vi "AIM 664 test Import Configuration File (Default Attributes).vi"(8 "error in (no error)":errorcluster, 11 "TestCase in":refnum<class "AIM 664 Import.lvclass">) -> (0 "error out":errorcluster, 3 "TestCase out":refnum<class "AIM 664 Import.lvclass">)   [LabVIEW 2020, in "AIM 664 Import.lvclass"]
uses:
  AIM 664 Import.lvclass
  Shared/Port Session Configuration.ctl
  Shared/board_setup.ctl
  Shared/port_configuration.ctl
  Shared/port_setup.ctl
  Shared/tx_udp_setup.ctl
  Shared/port_tx_udp_comm.ctl
  Shared/frame_parameter.ctl
  Shared/frame_parameter_definition.ctl
  <vilib>/NI/NI VeriStand Encoding and Decoding/Encoding.ctl
  Shared/port_tx_udp_sap.ctl
  Shared/rx_udp_setup.ctl
  Shared/port_rx_udp_comm.ctl
  Shared/port_rx_udp_sap.ctl
  <vilib>/addons/_JKI Toolkits/VI Tester/TestCase.llb/TestCase.lvclass
  <vilib>/NI/VeriStand Custom Device Testing Tools/VeriStandTestUtilities/VeriStandTestUtilities.lvlib
  Import/AIM ARINC 664 Import.lvlib
  <vilib>/NI/NI VeriStand Encoding and Decoding/Encoding and Decoding.lvlib
  C:/Program Files (x86)/National Instruments/LabVIEW 2020/vi.lib/addons/_JKI Toolkits/VI Tester/TestCase.llb/TestCase.lvclass
panel:
  out "x = y?":T1
  out "size(s)":i32
  out "index of element":i32[](array[numeric])
  out "logical AND 6":bool
  out "x = y? 2":bool[](array[boolean])
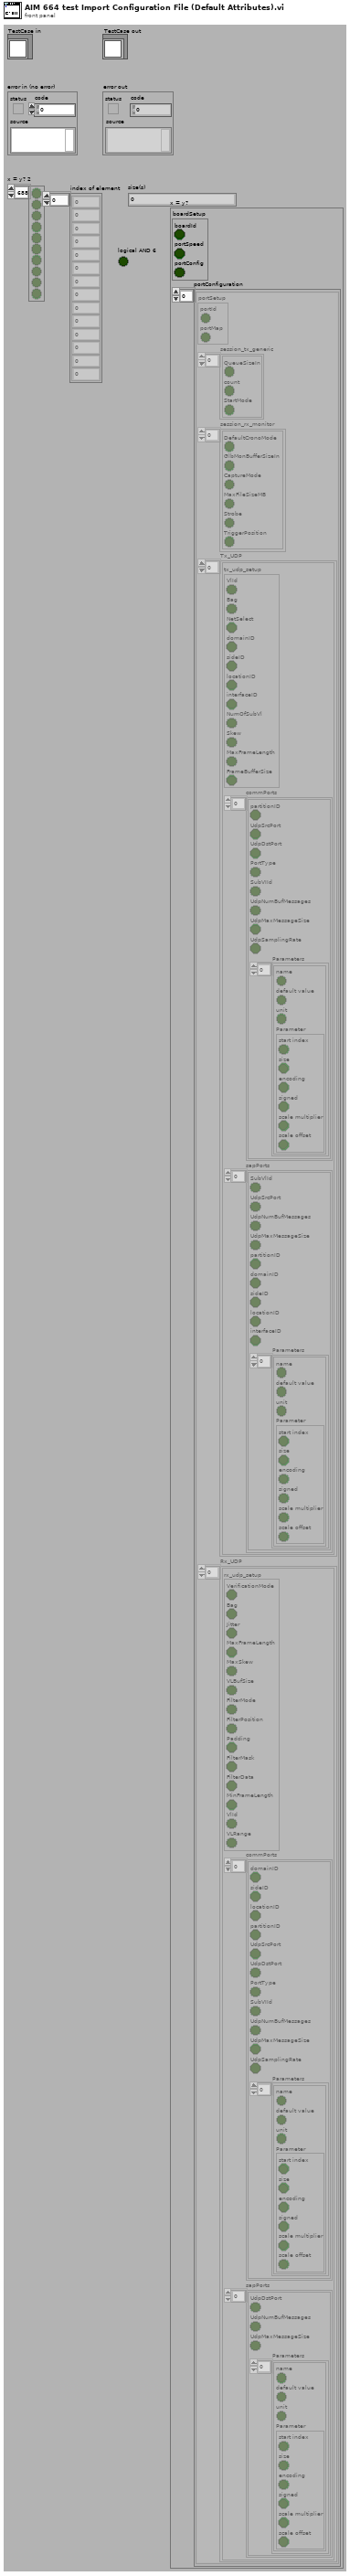
[diagram p1: front panel]
types:
  T1 = cluster{"boardSetup":cluster{"boardId":bool, "portSpeed":bool, "portConfig":bool}, "portConfiguration":cluster{"portSetup":cluster{"portId":bool, "portMap":bool}, "session_tx_generic":cluster{"QueueSizeIn":bool, "count":bool, "StartMode":bool}[], "session_rx_monitor":cluster{"DefaultCronoMode":bool, "GlbMonBufferSizeIn":bool, "CaptureMode":bool, "MaxFileSizeMB":bool, "Strobe":bool, "TriggerPosition":bool}[], "Tx_UDP":cluster{"tx_udp_setup":cluster{"VlId":bool, "Bag":bool, "NetSelect":bool, "domainID":bool, "sideID":bool, "locationID":bool, "interfaceID":bool, "NumOfSubVl":bool, "Skew":bool, "MaxFrameLength":bool, "FrameBufferSize":bool}, "commPorts":cluster{"partitionID":bool, "UdpSrcPort":bool, "UdpDstPort":bool, "PortType":bool, "SubVIId":bool, "UdpNumBufMessages":bool, "UdpMaxMessageSize":bool, "UdpSamplingRate":bool, "Parameters":cluster{"name":bool, "default value":bool, "unit":bool, "Parameter":cluster{"start index":bool, "size":bool, "encoding":bool, "signed":bool, "scale multiplier":bool, "scale offset":bool}}[]}[], "sapPorts":cluster{"SubVlId":bool, "UdpSrcPort":bool, "UdpNumBufMessages":bool, "UdpMaxMessageSize":bool, "partitionID":bool, "domainID":bool, "sideID":bool, "locationID":bool, "interfaceID":bool, "Parameters":cluster{"name":bool, "default value":bool, "unit":bool, "Parameter":cluster{"start index":bool, "size":bool, "encoding":bool, "signed":bool, "scale multiplier":bool, "scale offset":bool}}[]}[]}[], "Rx_UDP":cluster{"rx_udp_setup":cluster{"VerificationMode":bool, "Bag":bool, "Jitter":bool, "MaxFrameLength":bool, "MaxSkew":bool, "VLBufSize":bool, "FilterMode":bool, "FilterPosition":bool, "Padding":bool, "FilterMask":bool, "FilterData":bool, "MinFrameLength":bool, "VlId":bool, "VLRange":bool}, "commPorts":cluster{"domainID":bool, "sideID":bool, "locationID":bool, "partitionID":bool, "UdpSrcPort":bool, "UdpDstPort":bool, "PortType":bool, "SubVIId":bool, "UdpNumBufMessages":bool, "UdpMaxMessageSize":bool, "UdpSamplingRate":bool, "Parameters":cluster{"name":bool, "default value":bool, "unit":bool, "Parameter":cluster{"start index":bool, "size":bool, "encoding":bool, "signed":bool, "scale multiplier":bool, "scale offset":bool}}[]}[], "sapPorts":cluster{"UdpDstPort":bool, "UdpNumBufMessages":bool, "UdpMaxMessageSize":bool, "Parameters":cluster{"name":bool, "default value":bool, "unit":bool, "Parameter":cluster{"start index":bool, "size":bool, "encoding":bool, "signed":bool, "scale multiplier":bool, "scale offset":bool}}[]}[]}[]}[]}
  T2 = typedef "AIM ARINC 664 Import.lvlib/Port Session Configuration.ctl" = cluster{"boardSetup":T3, "portConfiguration":T4[]}
  T3 = typedef "AIM ARINC 664 Import.lvlib/board_setup.ctl" = cluster{"boardId":u32, "portSpeed":u32, "portConfig":u32}
  T4 = typedef "AIM ARINC 664 Import.lvlib/port_configuration.ctl" = cluster{"portSetup":T5, "session_tx_generic":cluster{"QueueSizeIn":u32, "count":i32, "StartMode":i32}[], "session_rx_monitor":cluster{"DefaultCronoMode":u32, "GlbMonBufferSizeIn":u32, "CaptureMode":u32, "MaxFileSizeMB":u32, "Strobe":u32, "TriggerPosition":u32}[], "Tx_UDP":cluster{"tx_udp_setup":T6, "commPorts":T7[], "sapPorts":T11[]}[], "Rx_UDP":cluster{"rx_udp_setup":T12, "commPorts":T13[], "sapPorts":T14[]}[]}
  T5 = typedef "AIM ARINC 664 Import.lvlib/port_setup.ctl" = cluster{"portId":u32, "portMap":u32}
  T6 = typedef "AIM ARINC 664 Import.lvlib/tx_udp_setup.ctl" = cluster{"VlId":i32, "Bag":i32, "NetSelect":i32, "domainID":u8, "sideID":u8, "locationID":u8, "interfaceID":u8, "NumOfSubVl":u16, "Skew":u32, "MaxFrameLength":u32, "FrameBufferSize":u32}
  T7 = typedef "AIM ARINC 664 Import.lvlib/port_tx_udp_comm.ctl" = cluster{"partitionID":u8, "UdpSrcPort":u16, "UdpDstPort":u16, "PortType":enum16{"FDX_UDP_SAMPLING", "FDX_UDP_QUEUING"}, "SubVIId":u32, "UdpNumBufMessages":u32, "UdpMaxMessageSize":u32, "UdpSamplingRate":u32, "Parameters":T8[]}
  T8 = typedef "AIM ARINC 664 Import.lvlib/frame_parameter.ctl" = cluster{"name":string, "default value":dbl, "unit":string, "Parameter":T9}
  T9 = typedef "AIM ARINC 664 Import.lvlib/frame_parameter_definition.ctl" = cluster{"start index":i32, "size":i32, "encoding":T10, "signed":bool, "scale multiplier":dbl, "scale offset":dbl}
  T10 = typedef "Encoding and Decoding.lvlib/Encoding.ctl" = enum16{"BNR", "BCD", "Discrete"}
  T11 = typedef "AIM ARINC 664 Import.lvlib/port_tx_udp_sap.ctl" = cluster{"SubVlId":u8, "UdpSrcPort":u16, "UdpNumBufMessages":u32, "UdpMaxMessageSize":u32, "partitionID":u8, "domainID":u8, "sideID":u8, "locationID":u8, "interfaceID":u8, "Parameters":T8[]}
  T12 = typedef "AIM ARINC 664 Import.lvlib/rx_udp_setup.ctl" = cluster{"VerificationMode":u32, "Bag":u32, "Jitter":u32, "MaxFrameLength":u32, "MaxSkew":u32, "VLBufSize":u32, "FilterMode":u32, "FilterPosition":u32, "Padding":u32, "FilterMask":u32, "FilterData":u32, "MinFrameLength":u32, "VlId":u16, "VLRange":u32}
  T13 = typedef "AIM ARINC 664 Import.lvlib/port_rx_udp_comm.ctl" = cluster{"domainID":u8, "sideID":u8, "locationID":u8, "partitionID":u8, "UdpSrcPort":u16, "UdpDstPort":u16, "PortType":enum16{"FDX_UDP_SAMPLING", "FDX_UDP_QUEUING"}, "SubVIId":u32, "UdpNumBufMessages":u32, "UdpMaxMessageSize":u32, "UdpSamplingRate":u32, "Parameters":T8[]}
  T14 = typedef "AIM ARINC 664 Import.lvlib/port_rx_udp_sap.ctl" = cluster{"UdpDstPort":u16, "UdpNumBufMessages":u32, "UdpMaxMessageSize":u32, "Parameters":T8[]}
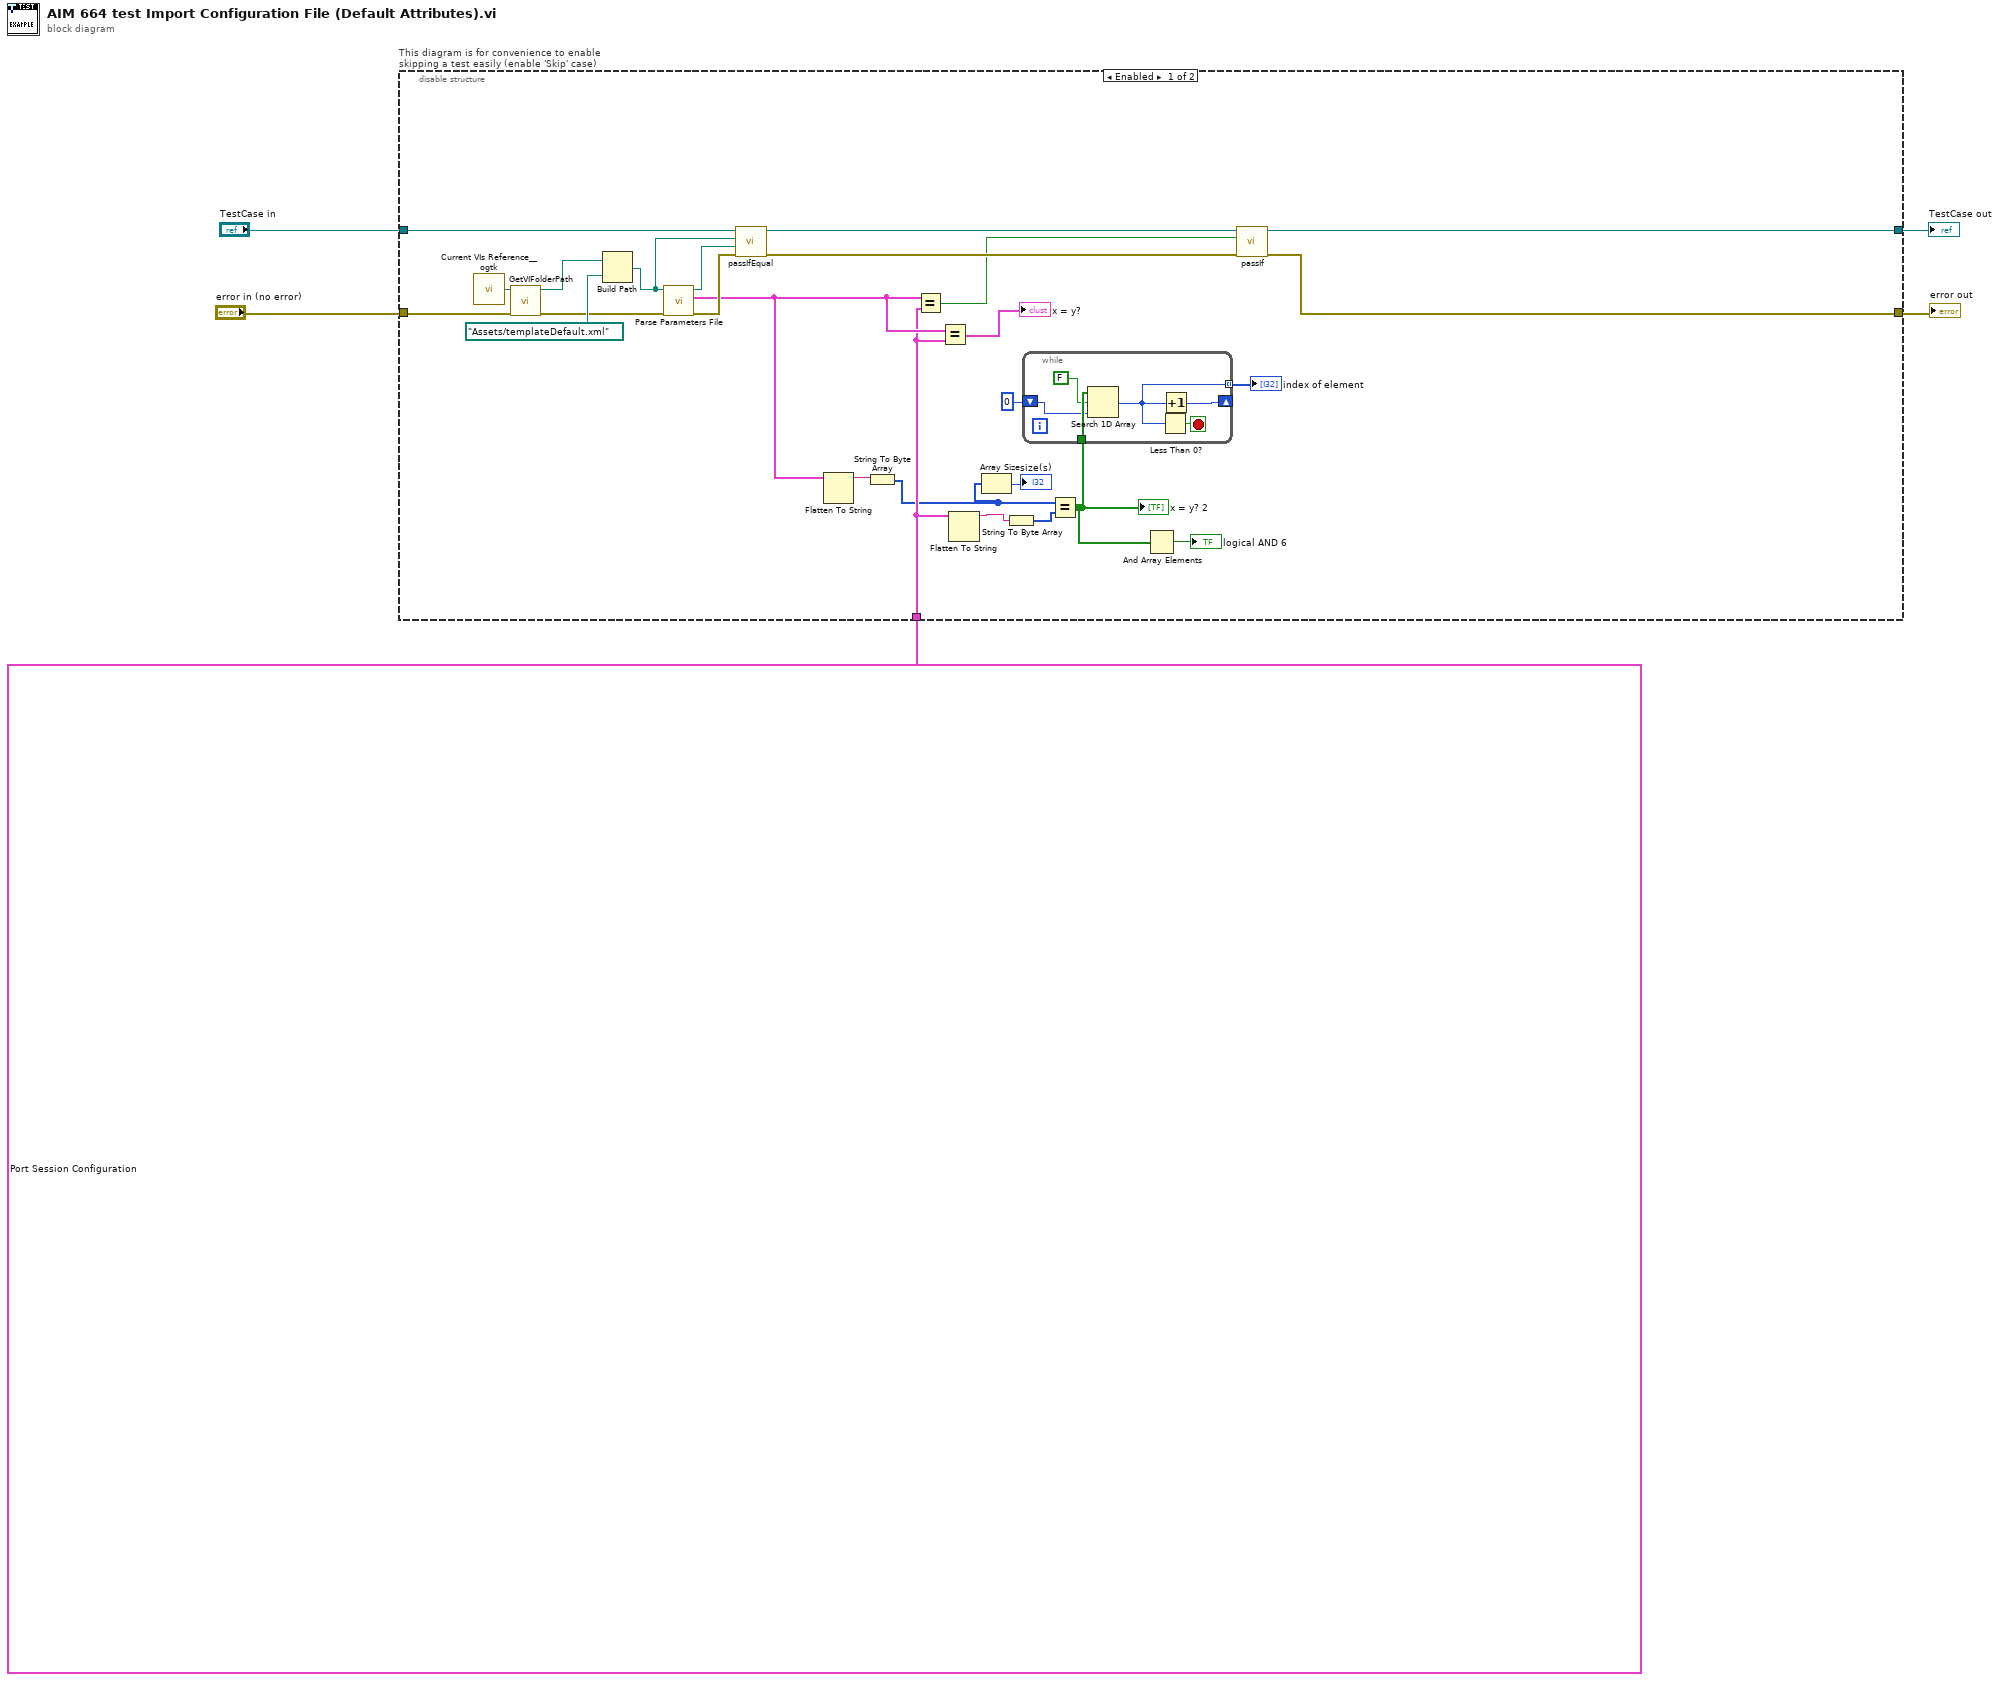
[diagram p0: block diagram]
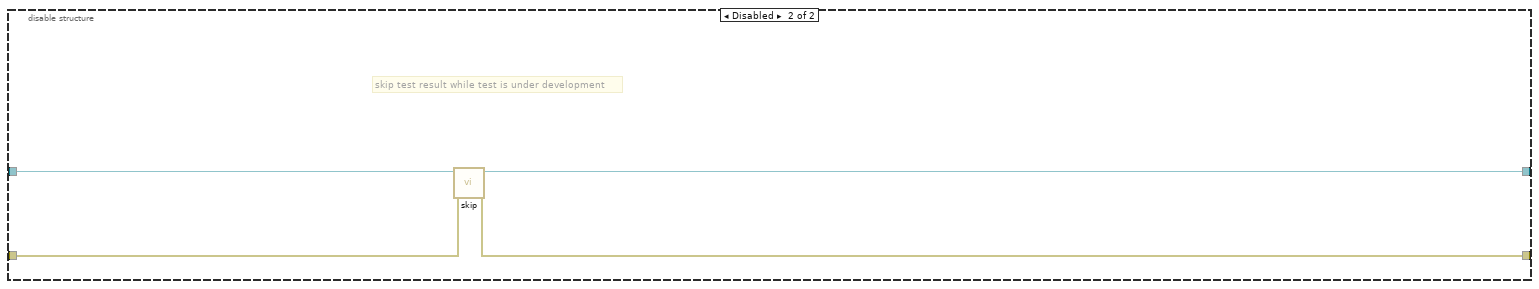
[diagram p2: hidden frame]
diagram:
  n1 = disable-structure "This diagram is for convenience to enable skipping a test easily (enable 'Skip' case)" shown="Enabled" {
    disable-tunnel: "TestCase in" -> [w24 w41]
    disable-tunnel: [w26 w39] -> w2
    disable-tunnel: [w25 w40] -> w4
    disable-tunnel: "error in (no error)" -> [w29 w38]
    disable-tunnel: T2 {"boardSetup"={"boardId"=0, "portSpeed"=0, "portConfig"=0}, "portConfiguration"=[{"portSetup"={"portId"=0, "portMap"=0}, "session_tx_generic"=[{"QueueSizeIn"=0, "count"=0, "StartMode"=1}], "session_rx_monitor"=[{"DefaultCronoMode"=1, "GlbMonBufferSizeIn"=0, "CaptureMode"=1, "MaxFileSizeMB"=1, "Strobe"=0, "TriggerPosition"=0}], "Tx_UDP"=[], "Rx_UDP"=[]}, {"portSetup"={"portId"=1, "portMap"=0}, "session_tx_generic"=[], "session_rx_monitor"=[], "Tx_UDP"=[{"tx_udp_setup"={"VlId"=0, "Bag"=1, "NetSelect"=2, "domainID"=0, "sideID"=0, "locationID"=0, "interfaceID"=0, "NumOfSubVl"=1, "Skew"=0, "MaxFrameLength"=0, "FrameBufferSize"=0}, "commPorts"=[{"partitionID"=0, "UdpSrcPort"=0, "UdpDstPort"=0, "PortType"=enum."FDX_UDP_SAMPLING", "SubVIId"=1, "UdpNumBufMessages"=0, "UdpMaxMessageSize"=0, "UdpSamplingRate"=1, "Parameters"=[{"name"="Param 0", "default value"=0.0, "unit"="", "Parameter"={"start index"=0, "size"=0, "encoding"=enum."BNR", "signed"=FALSE, "scale multiplier"=0.0, "scale offset"=0.0}}, {"name"="Param 1", "default value"=0.0, "unit"="", "Parameter"={"start index"=0, "size"=0, "encoding"=enum."BNR", "signed"=FALSE, "scale multiplier"=0.0, "scale offset"=0.0}}, {"name"="Param 2", "default value"=0.0, "unit"="", "Parameter"={"start index"=0, "size"=0, "encoding"=enum."BNR", "signed"=FALSE, "scale multiplier"=0.0, "scale offset"=0.0}}]}], "sapPorts"=[{"SubVlId"=1, "UdpSrcPort"=0, "UdpNumBufMessages"=0, "UdpMaxMessageSize"=0, "partitionID"=0, "domainID"=0, "sideID"=0, "locationID"=0, "interfaceID"=0, "Parameters"=[{"name"="Param 0", "default value"=0.0, "unit"="", "Parameter"={"start index"=0, "size"=0, "encoding"=enum."BNR", "signed"=FALSE, "scale multiplier"=0.0, "scale offset"=0.0}}, {"name"="Param 1", "default value"=0.0, "unit"="", "Parameter"={"start index"=0, "size"=0, "encoding"=enum."BNR", "signed"=FALSE, "scale multiplier"=0.0, "scale offset"=0.0}}, {"name"="Param 2", "default value"=0.0, "unit"="", "Parameter"={"start index"=0, "size"=0, "encoding"=enum."BNR", "signed"=FALSE, "scale multiplier"=0.0, "scale offset"=0.0}}]}]}], "Rx_UDP"=[{"rx_udp_setup"={"VerificationMode"=0, "Bag"=1, "Jitter"=1, "MaxFrameLength"=0, "MaxSkew"=0, "VLBufSize"=0, "FilterMode"=0, "FilterPosition"=0, "Padding"=0, "FilterMask"=0, "FilterData"=0, "MinFrameLength"=0, "VlId"=0, "VLRange"=0}, "commPorts"=[{"domainID"=0, "sideID"=0, "locationID"=0, "partitionID"=0, "UdpSrcPort"=0, "UdpDstPort"=0, "PortType"=enum."FDX_UDP_SAMPLING", "SubVIId"=0, "UdpNumBufMessages"=1, "UdpMaxMessageSize"=0, "UdpSamplingRate"=0, "Parameters"=[{"name"="Param 0", "default value"=0.0, "unit"="", "Parameter"={"start index"=0, "size"=0, "encoding"=enum."BNR", "signed"=FALSE, "scale multiplier"=0.0, "scale offset"=0.0}}, {"name"="Param 1", "default value"=0.0, "unit"="", "Parameter"={"start index"=0, "size"=0, "encoding"=enum."BNR", "signed"=FALSE, "scale multiplier"=0.0, "scale offset"=0.0}}]}], "sapPorts"=[{"UdpDstPort"=0, "UdpNumBufMessages"=0, "UdpMaxMessageSize"=0, "Parameters"=[{"name"="Param 0", "default value"=0.0, "unit"="", "Parameter"={"start index"=0, "size"=0, "encoding"=enum."BNR", "signed"=FALSE, "scale multiplier"=0.0, "scale offset"=0.0}}, {"name"="Param 1", "default value"=0.0, "unit"="", "Parameter"={"start index"=0, "size"=0, "encoding"=enum."BNR", "signed"=FALSE, "scale multiplier"=0.0, "scale offset"=0.0}}]}]}]}]} ("board configuration") -> [w16 _]
    frame Enabled {
      n2 = call <userlib>:"Current VIs Reference__ogtk.vi"() -> ("Current VI's reference"=w31:refnum<vi>)  [unwired: 5 in]
      n3 = call <vilib>:"GetVIFolderPath.vi"("error in (no error)"=w29, "VI Reference in"=w31) -> ("error out"=w27:errorcluster, "VI Folder Path out"=w30:path)  [unwired: 8 in]
      n4 = Build Path(base path=w30, name or relative path=path "Assets/templateDefault.xml") -> (appended path=w21:path)
      n5 = call "Parse Parameters File.vi"("error in"=w27, "path to XML document"=w21) -> ("error out"=w22:errorcluster, "board configuration"=w17:T2, "path to XML document out"=w20:path)  [unwired: 7 in]
      n6 = call-dynamic "passIfEqual.vi"("error in (no error)"=w22, "y"=w20, "x"=w21, "TestCase in"=w24) -> ("error out"=w19:errorcluster, "TestCase out"=w23:refnum<class "AIM 664 Import.lvclass">)  [unwired: 6 in]
      n7 = Flatten To String(anything=w17) -> (data string=w15:string)  [unwired: 3 in, 2 out]
      n8 = String To Byte Array(string=w15) -> (unsigned byte array=w10:u8[])
      n9 = Equal?(x=w17, y=w16) -> (x = y?=w18:bool)
      n10 = Equal?(x=w17, y=w16) -> (x = y?=→"x = y?":T1)
      n11 = Flatten To String(anything=w16) -> (data string=w14:string)  [unwired: 3 in, 2 out]
      n12 = Array Size(array=w10) -> (size(s)=→"size(s)":i32)
      n13 = String To Byte Array(string=w14) -> (unsigned byte array=w13:u8[])
      n14 = Equal?(x=w10, y=w13) -> (x = y?=w11:bool[])
      "x = y? 2" <- w11
      n15 = while {
        tunnel: w11 -> [w37]
        tunnel: [w34] -> w8 mode=indexing
        shift-right: [w32] -> _
        shift-left: 0 ("index of element") -> [w33]
        stop <- w35 stop-if-true
        n16 = Search 1D Array(1D array=w37, element=FALSE ("logical AND 6"), start index (0)=w33) -> (index of element=w34:i32)
        n17 = Less Than 0?(x=w34) -> (x < 0?=w35:bool)
        n18 = Increment(x=w34) -> (x+1=w32:i32)
      }
      "index of element" <- w8
      n19 = And Array Elements(Boolean array=w11) -> (logical AND=→"logical AND 6":bool)
      n20 = call-dynamic "passIf.vi"("error in (no error)"=w19, "pass"=w18, "TestCase in"=w23) -> ("error out"=w25:errorcluster, "TestCase out"=w26:refnum<class "AIM 664 Import.lvclass">)  [unwired: 7 in]
    }
    frame Disabled {
      # "skip test result while test is under development"
      n21 = call <vilib>:"skip.vi"("error in (no error)"=w38, "TestCase in"=w41) -> ("error out"=w40:errorcluster, "TestCase out"=w39:refnum<class "AIM 664 Import.lvclass">)  [unwired: 8 in]
    }
  }
  "error out" <- w4
  "TestCase out" <- w2
